vi "VLC Viewer my.vi"() -> ()   [LabVIEW 2016]
panel:
  out "2D Picture":picture
  in  "uri":string="rtsp://admin:admin@192.168.1.108/cam/realmonitor?channel=1&subtype=1"
  out "PlaylistIndex":i32
  in  "Clear":bool
  out "PlaylistCount":i32
  in  "load":bool
  in  "exit":bool
  in  "stop":bool
  in  "pause":bool
  in  "play":bool
  out "error out":errorcluster
  in  "VLCPlugin2":refnum<k7>(container)
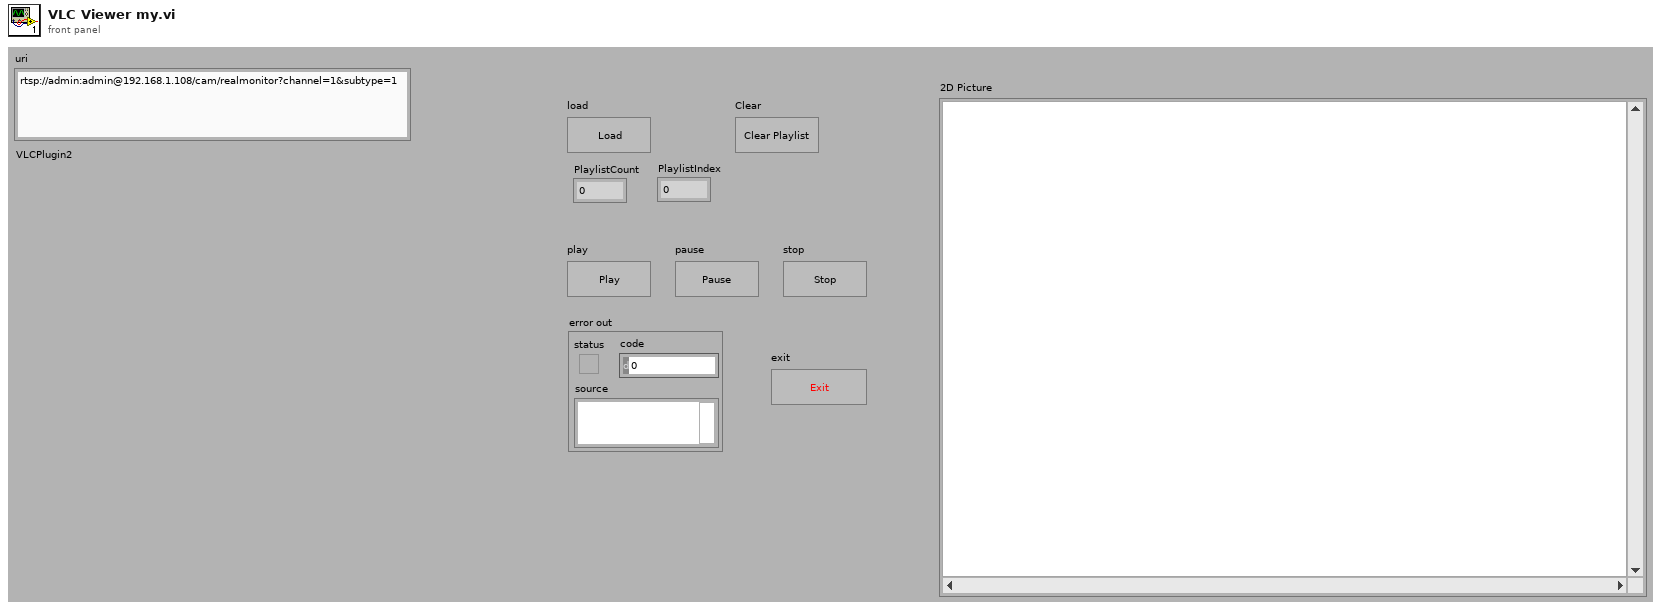
[diagram p1: front panel]
types:
  T1 = typedef "imagedata.ctl" = cluster{"image type":i32, "image depth":i32, "image":u8[], "mask":u8[], "colors":u32[], "Rectangle":cluster{"left":i16, "top":i16, "right":i16, "bottom":i16}}
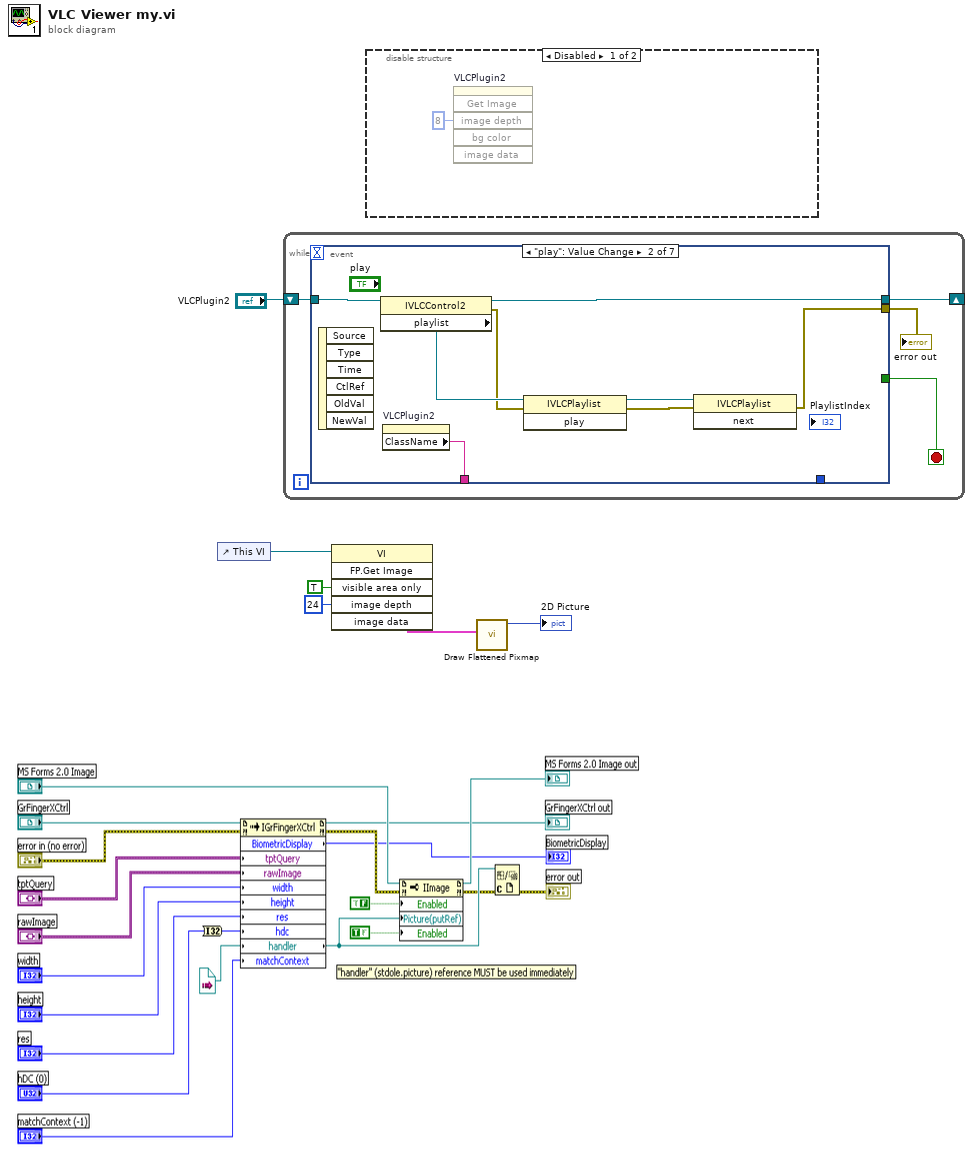
[diagram p0: block diagram]
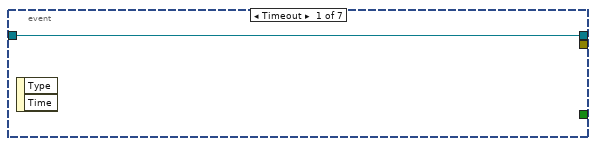
[diagram p3: hidden frame]
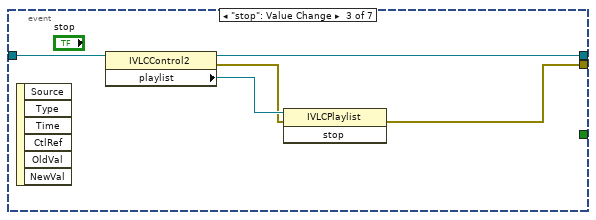
[diagram p4: hidden frame]
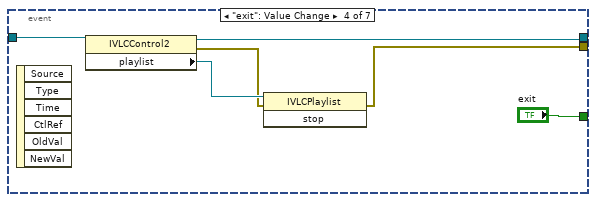
[diagram p5: hidden frame]
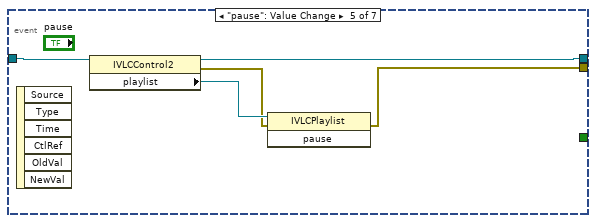
[diagram p6: hidden frame]
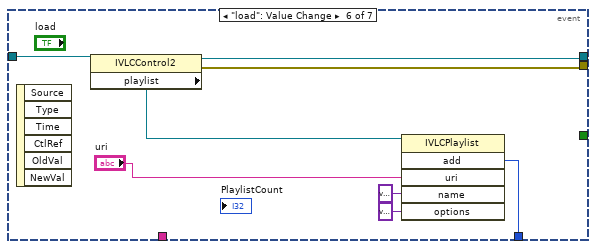
[diagram p7: hidden frame]
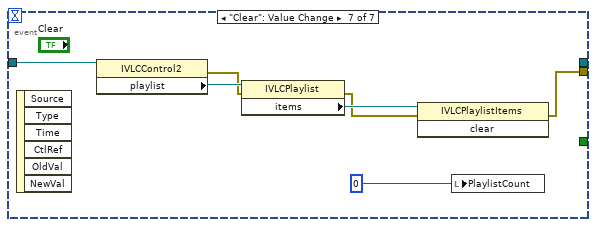
[diagram p8: hidden frame]
diagram:
  n1 = control-ref of="This VI"() -> (w5:refnum<vi>)
  n2 = while {
    shift-right: [w7] -> _
    shift-left: "VLCPlugin2" -> [w10]
    stop <- w8 stop-if-true
    n3 = event shown="[1] \"play\": Value Change" {
      selector: _ -> [_ _ _ _ _ _ _]
      dyn-events: _ -> [_ _ _ _ _ _ _]
      timeout: _ -> [_ _ _ _ _ _ _]
      tunnel: w10 -> [w11 w19 w24 w27 w33 w42 w50]
      tunnel: [_ w15 w20 w25 w32 w43 w45] -> w9
      tunnel: [_ _ _ "exit" _ _ _] -> w8
      tunnel: [w11 w12 w22 w26 w31 w41 _] -> w7
      tunnel: [_ _ _ _ _ w40 _] -> _
      tunnel: [_ w14 _ _ _ _ _] -> _
      event Timeout {
        n4 = event-data() -> ()  [unwired: 3 out]
      }
      event "play": Value Change {
        n5 = event-data() -> ()  [unwired: 7 out]
        n6 = property class="IVLCControl2"(reference=w19) -> (reference out=w12:refnum<k7>, error out=w17:errorcluster, "playlist"=w18:refnum<k7>)  [unwired: 1 in]
        n7 = property on="VLCPlugin2" class="AXCont"() -> ("ClassName"=w14:string)  [unwired: 2 in, 2 out]
        n8 = invoke class="IVLCPlaylist" method="play"(reference=w18, error in=w17) -> (reference out=w13:refnum<k7>, error out=w16:errorcluster)  [unwired: 1 in, 1 out]
        n9 = invoke class="IVLCPlaylist" method="next"(reference=w13, error in=w16) -> (error out=w15:errorcluster)  [unwired: 1 in, 2 out]
      }
      event "stop": Value Change {
        n10 = event-data() -> ()  [unwired: 7 out]
        n11 = property class="IVLCControl2"(reference=w24) -> (reference out=w22:refnum<k7>, error out=w21:errorcluster, "playlist"=w23:refnum<k7>)  [unwired: 1 in]
        n12 = invoke class="IVLCPlaylist" method="stop"(reference=w23, error in=w21) -> (error out=w20:errorcluster)  [unwired: 1 in, 2 out]
      }
      event "exit": Value Change {
        n13 = event-data() -> ()  [unwired: 7 out]
        n14 = property class="IVLCControl2"(reference=w27) -> (reference out=w26:refnum<k7>, error out=w28:errorcluster, "playlist"=w29:refnum<k7>)  [unwired: 1 in]
        n15 = invoke class="IVLCPlaylist" method="stop"(reference=w29, error in=w28) -> (error out=w25:errorcluster)  [unwired: 1 in, 2 out]
      }
      event "pause": Value Change {
        n16 = event-data() -> ()  [unwired: 7 out]
        n17 = property class="IVLCControl2"(reference=w33) -> (reference out=w31:refnum<k7>, error out=w34:errorcluster, "playlist"=w35:refnum<k7>)  [unwired: 1 in]
        n18 = invoke class="IVLCPlaylist" method="pause"(reference=w35, error in=w34) -> (error out=w32:errorcluster)  [unwired: 1 in, 2 out]
      }
      event "load": Value Change {
        n19 = event-data() -> ()  [unwired: 7 out]
        n20 = property class="IVLCControl2"(reference=w42) -> (reference out=w41:refnum<k7>, error out=w43:errorcluster, "playlist"=w39:refnum<k7>)  [unwired: 1 in]
        n21 = invoke class="IVLCPlaylist" method="add"(reference=w39, "uri"="uri", "name"=variant, "options"=variant) -> ("add"=w40:i32)  [unwired: 2 in, 5 out]
      }
      event "Clear": Value Change {
        n22 = event-data() -> ()  [unwired: 7 out]
        n23 = property class="IVLCControl2"(reference=w50) -> (error out=w48:errorcluster, "playlist"=w49:refnum<k7>)  [unwired: 1 in, 1 out]
        n24 = property class="IVLCPlaylist"(reference=w49, error in=w48) -> (error out=w46:errorcluster, "items"=w47:refnum<k7>)  [unwired: 1 out]
        n25 = invoke class="IVLCPlaylistItems" method="clear"(reference=w47, error in=w46) -> (error out=w45:errorcluster)  [unwired: 1 in, 2 out]
        n26 = local write "PlaylistCount"(0 ("PlaylistCount")) -> ()
      }
    }
    "error out" <- w9
  }
  n27 = invoke class="VI" method="FP.Get Image"(reference=w5, "visible area only"=TRUE ("Visible Area Only"), "image depth"=24 ("Image Depth")) -> ("image data"=w3:T1)  [unwired: 3 in, 5 out]
  n28 = disable-structure shown="Disabled" {
    frame Disabled {
      n29 = invoke on="VLCPlugin2" class="AXCont" method="Get Image"("image depth"=8 ("Image Depth")) -> ()  [unwired: 5 in, 6 out]
    }
    frame Enabled {
    }
  }
  n30 = call <vilib>:"Draw Flattened Pixmap.vi"("image data"=w3) -> ("new picture"=→"2D Picture":picture)  [unwired: 8 in]
